vi "Save_SpectralGateSweep.vi"(0 "Refnum in":refnum<k34>, 1 "Integrated Emission":dbl[](array[numeric]), 2 "Capture number":i32, 3 "Integration Center WL":dbl=770.0 format="%#_13g", 5 "New file":bool=TRUE, 7 "Image":dbl[][](array[numeric]), 11 "error in (no error)":errorcluster, 12 "Gate Delay array":dbl[](array[numeric]), 13 "Wavelength Array":dbl[](array[numeric]), 14 "WL width":dbl=5.0 format="%#_13g") -> (4 "Refnum out":refnum<k34>, 15 "error out":errorcluster)   [LabVIEW 2018]
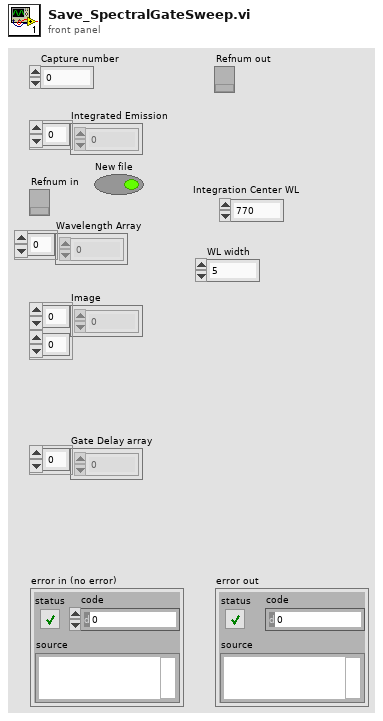
[diagram p1: front panel]
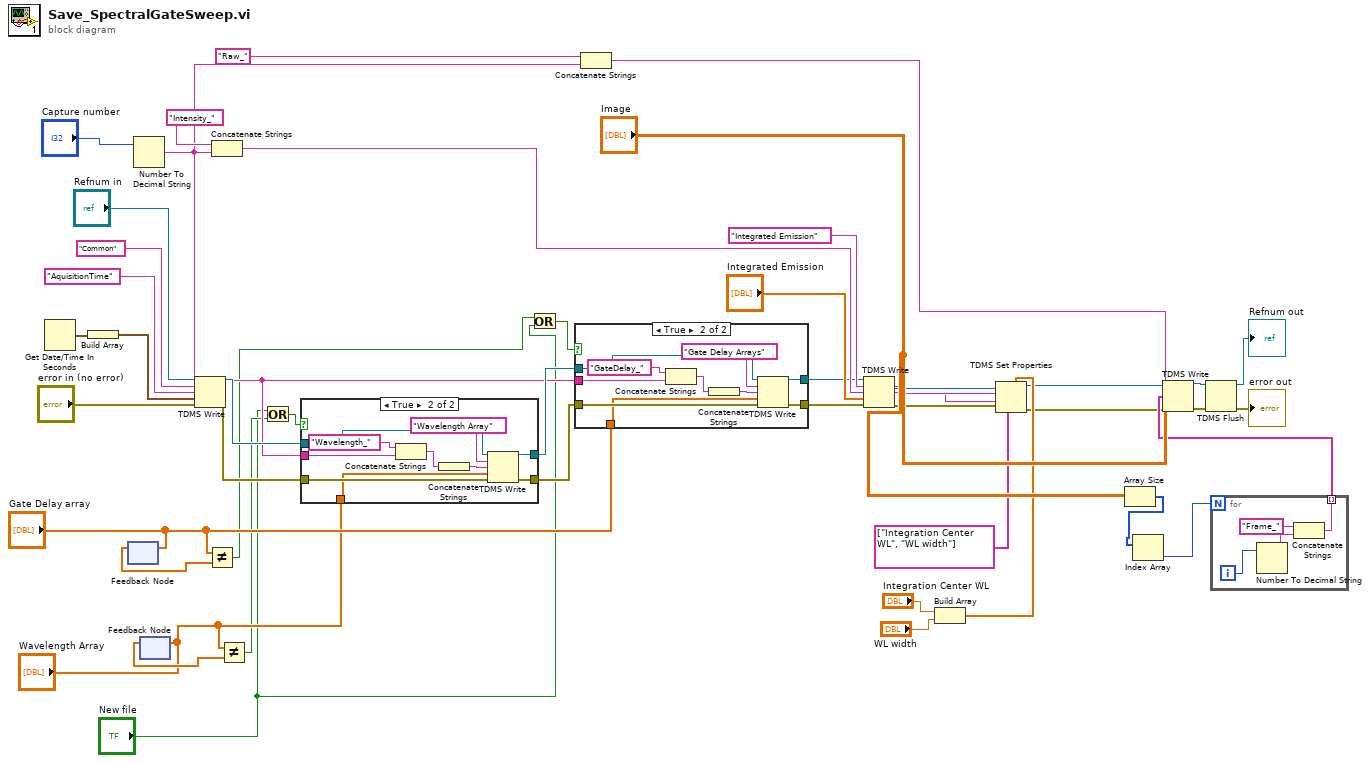
[diagram p0: block diagram]
diagram:
  n1 = Get Date/Time In Seconds() -> (seconds since 1Jan1904=w28:timestamp)
  n2 = Build Array(w28) -> (w32:timestamp[])
  n3 = feedback #1() -> (w30:dbl[])  [unwired: 1 in]
  n4 = feedback-in #1("Gate Delay array") -> ()
  n5 = Number To Decimal String(number="Capture number") -> (decimal integer string=w16:string)  [unwired: 1 in]
  n6 = feedback #2() -> (w18:dbl[])  [unwired: 1 in]
  n7 = feedback-in #2("Wavelength Array") -> ()
  n8 = TDMS Write(0:"Refnum in", 5:"Common" ("group name in (Untitled)"), 7:"AquisitionTime", 9:w32, 11:"error in (no error)") -> (4:w22:refnum<k34>, 15:w21:errorcluster)  [unwired: 1 in, 2 out]
  n9 = Not Equal?(x="Gate Delay array", y=w30) -> (x != y?=w12:bool)
  n10 = Concatenate Strings("Intensity_" ("group name in (Untitled)"), w16) -> (w37:string)
  n11 = Not Equal?(x="Wavelength Array", y=w18) -> (x != y?=w15:bool)
  n12 = Or(x="New file", y=w15) -> (x .or. y?=w14:bool)
  n13 = case shown="True" w14 {
    tunnel: w22 -> [w49 w59]
    tunnel: w21 -> [w48 w58]
    tunnel: [w49 w57] -> w20
    tunnel: [w48 w56] -> w19
    tunnel: "Wavelength Array" -> [_ w53]
    tunnel: w16 -> [_ w50]
    frame False {
    }
    frame True {
      n14 = Concatenate Strings("Wavelength_" ("string"), w50) -> (w52:string)
      n15 = Concatenate Strings(w52) -> (w54:string)
      n16 = TDMS Write(0:w59, 5:"Wavelength Array" ("group name in (Untitled)"), 7:w54, 9:w53, 11:w58) -> (4:w57:refnum<k34>, 15:w56:errorcluster)  [unwired: 1 in, 2 out]
    }
  }
  n17 = Or(x=w12, y="New file") -> (x .or. y?=w11:bool)
  n18 = case shown="True" w11 {
    tunnel: w20 -> [w61 w71]
    tunnel: w19 -> [w60 w70]
    tunnel: [w61 w69] -> w34
    tunnel: [w60 w68] -> w35
    tunnel: "Gate Delay array" -> [_ w65]
    tunnel: w16 -> [_ w62]
    frame False {
    }
    frame True {
      n19 = Concatenate Strings("GateDelay_" ("string"), w62) -> (w64:string)
      n20 = Concatenate Strings(w64) -> (w66:string)
      n21 = TDMS Write(0:w71, 5:"Gate Delay Arrays" ("group name in (Untitled)"), 7:w66, 9:w65, 11:w70) -> (4:w69:refnum<k34>, 15:w68:errorcluster)  [unwired: 1 in, 2 out]
    }
  }
  n22 = Concatenate Strings("Raw_" ("group name in (Untitled)"), w16) -> (w41:string)
  n23 = TDMS Write(0:w34, 5:"Integrated Emission" ("group name in (Untitled)"), 7:w37, 9:"Integrated Emission", 11:w35) -> (4:w9:refnum<k34>, 6:w8:string, 8:w7:string, 15:w10:errorcluster)  [unwired: 1 in]
  n24 = Build Array("Integration Center WL", "WL width") -> (w3:dbl[])
  n25 = TDMS Set Properties(5:w3, 7:string[] ["Integration Center WL", "WL width"] ("property names"), 8:w10, 9:w7, 10:w8, 11:w9) -> (0:w1:errorcluster, 3:w2:refnum<k34>)  [unwired: 2 out]
  n26 = Array Size(array="Image") -> (size(s)=w26:i32[])
  n27 = Index Array(array=w26) -> (element=w25:i32)  [unwired: 1 in]
  n28 = for {
    N: w25 -> [_]
    tunnel: [w72] -> w24 mode=indexing
    i -> [w75]
    n29 = Number To Decimal String(number=w75) -> (decimal integer string=w74:string)  [unwired: 1 in]
    n30 = Concatenate Strings("Frame_" ("string"), w74) -> (w72:string)
  }
  n31 = TDMS Write(0:w2, 5:w41, 7:w24, 9:"Image", 11:w1) -> (4:w38:refnum<k34>, 15:w39:errorcluster)  [unwired: 1 in, 2 out]
  n32 = TDMS Flush(4:w39, 7:w38) -> (0:→"error out":errorcluster, 3:→"Refnum out":refnum<k34>)
